vi "Breathalyze(SubVI).vi"(8 "error in (no error)":errorcluster, 10 "Str Refnum":refnum<vi>, 11 "LINX Ref":T1) -> (0 "error out":errorcluster, 2 "Average of array":dbl, 3 "LINX Resource":T1)   [LabVIEW 2014]
uses:
  <vilib>/MakerHub/LINX/Private/Type Defs/LINX Ref.ctl
  <vilib>/MakerHub/LINX/Private/Type Defs/Platform.ctl
  <vilib>/MakerHub/LINX/Private/Type Defs/Interface.ctl
  <vilib>/MakerHub/LINX/Private/Device/Type Defs/LINX Device Config.ctl
  <vilib>/MakerHub/LINX/Private/Device/Type Defs/TCP Config.ctl
  <vilib>/MakerHub/LINX/Private/Device/Type Defs/Channels.ctl
  BreathalyzeStates(Typedef).ctl
  <vilib>/MakerHub/LINX/Public/Peripherals/Analog/Analog Read 1 Chan.vi
  <vilib>/MakerHub/LINX/LMH-LINX.lvlib
  <vilib>/MakerHub/LINX/Private/Device/Device.lvlib
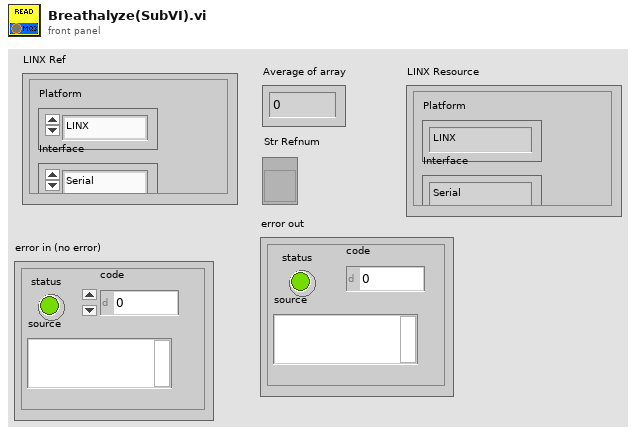
[diagram p1: front panel]
types:
  T1 = typedef "LMH-LINX.lvlib/LINX Ref.ctl" = cluster{"Platform":T2, "Interface":T3, "LINX Device Config":T4}
  T2 = typedef "LMH-LINX.lvlib/Platform.ctl" = enum16{"LINX", "myRIO"}
  T3 = typedef "LMH-LINX.lvlib/Interface.ctl" = enum16{"Serial", "TCP"}
  T4 = typedef "LMH-LINX.lvlib/Device.lvlib/LINX Device Config.ctl" = cluster{"Interface":T3, "COM Port":refnum<visa-resource-name>, "TCP Configuration":T5, "Device Family":u8, "Device ID":u8, "Device Name":string, "TCP Ref":refnum<k5>, "Channels":T6}
  T5 = typedef "LMH-LINX.lvlib/Device.lvlib/TCP Config.ctl" = cluster{"IP Address":string, "Port":u16}
  T6 = typedef "LMH-LINX.lvlib/Channels.ctl" = cluster{"DI":u8[], "DO":u8[], "AI":u8[], "AO":u8[], "PWM":u8[], "QE":u8[], "UART":u8[], "I2C 2":u8[], "SPI":u8[], "CAN":u8[], "Servo":u8[], "AI Ref (V)":dbl, "AO Ref (V)":dbl, "AO Resolution (Bits)":u8}
  T7 = typedef "BreathalyzeStates(Typedef).ctl" = enum16{"Prompt User", "Read Analog"}
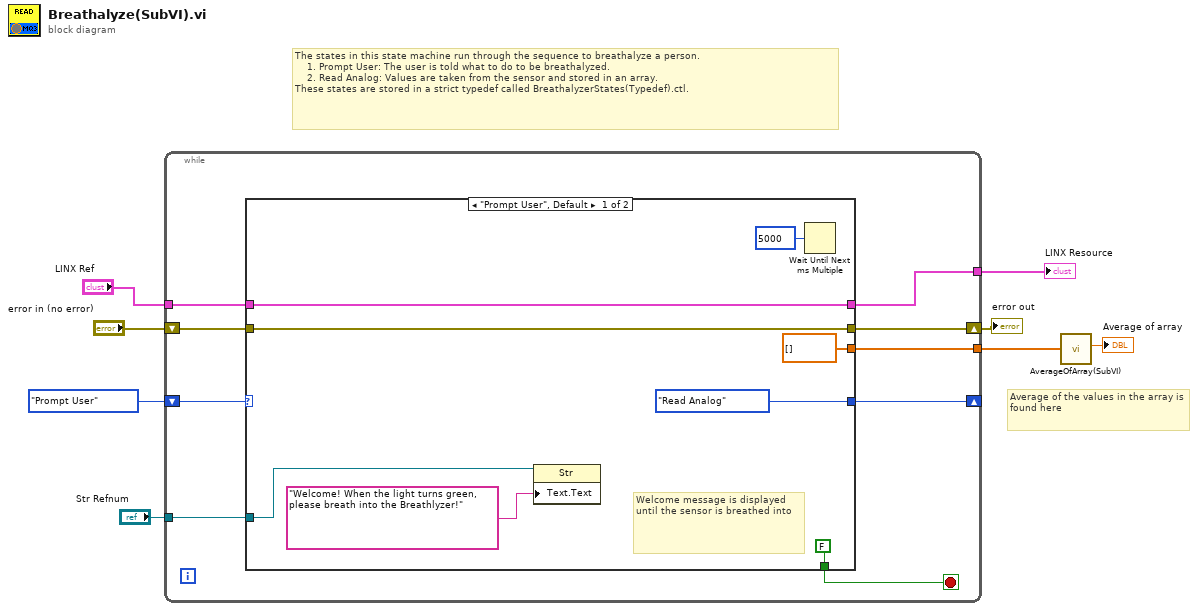
[diagram p0: block diagram]
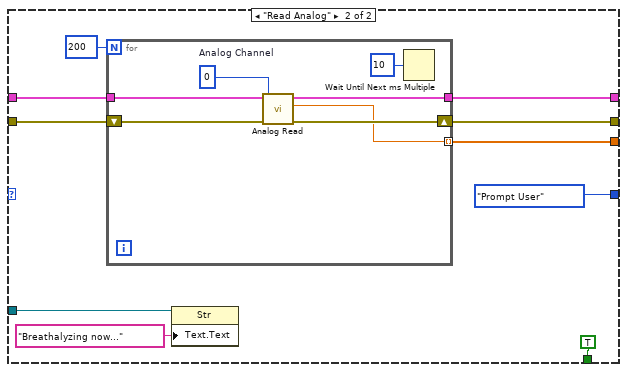
[diagram p2: hidden frame]
diagram:
  # "Average of the values in the array is found here"
  # "The states in this state machine run through the sequence to breathalyze a person.\n    1. Prompt User: The user is told what to do to be breathalyzed.\n    2. Read Analog: Values are taken from the sensor and stored in an array.\nThese states are stored in a strict typedef called BreathalyzerStates(Typedef).ctl."
  n1 = while {
    tunnel: "Str Refnum" -> [w16]
    shift-right: [w15] -> _
    shift-left: BreathalyzeStates(Typedef)."Prompt User" -> [w17]
    tunnel: "LINX Ref" -> [w14]
    tunnel: [w10] -> w3
    tunnel: [w9] -> w1
    shift-right: [w12] -> w4
    shift-left: "error in (no error)" -> [w13]
    stop <- w11 stop-if-true
    n2 = case shown="\"Prompt User\", Default" w17 {
      tunnel: w16 -> [w25 w33]
      tunnel: [BreathalyzeStates(Typedef)."Read Analog" BreathalyzeStates(Typedef)."Prompt User"] -> w15
      tunnel: w14 -> [w19 w32]
      tunnel: w13 -> [w18 w31]
      tunnel: [w18 w30] -> w12
      tunnel: [FALSE TRUE] -> w11
      tunnel: [dbl[] [] w27] -> w10
      tunnel: [w19 w26] -> w9
      frame "Prompt User", Default {
        # "Welcome message is displayed until the sensor is breathed into"
        n3 = property class="Str"(reference=w25, "Text.Text"="Welcome! When the light turns green, please breath into the Breathlyzer!") -> ()  [unwired: 1 in, 2 out]
        n4 = Wait Until Next ms Multiple(millisecond multiple=u32 5000) -> ()  [unwired: 1 out]
      }
      frame "Read Analog" {
        n5 = for {
          N: 200 -> [_]
          tunnel: w32 -> [w42]
          shift-right: [w40] -> w30
          shift-left: w31 -> [w41]
          tunnel: [w37] -> w27 mode=indexing
          tunnel: [w36] -> w26
          w39 = u8 0  # Analog Channel
          n6 = call-poly <vilib>:"Analog Read.vi"("Error In"=w41, "Analog Channel"=w39, "LINX Resource"=w42) -> ("Error Out"=w40:errorcluster, "AI Value"=w37:dbl, "LINX Resource"=w36:T1)  [unwired: 5 in, 1 out]
          n7 = Wait Until Next ms Multiple(millisecond multiple=u32 10) -> ()  [unwired: 1 out]
        }
        n8 = property class="Str"(reference=w33, "Text.Text"="Breathalyzing now...") -> ()  [unwired: 1 in, 2 out]
      }
    }
  }
  "error out" <- w4
  "LINX Resource" <- w1
  n9 = call "AverageOfArray(SubVI).vi"("Array"=w3) -> ("Average of array"=→"Average of array":dbl)  [unwired: 10 in]
